vi "InitAll.vi"() -> (0 "error IO":errorcluster caption="error out")   [LabVIEW 2018]
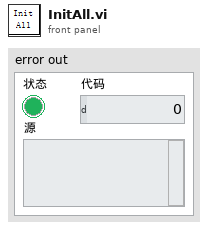
[diagram p1: front panel]
types:
  T1 = cluster{"Selected Index []":i32[], "Selected Items":string[]}
  T2 = enum16{"功率测量", "能量测量", "光谱测量", "时间波形", "偏振测量", "近远场"}
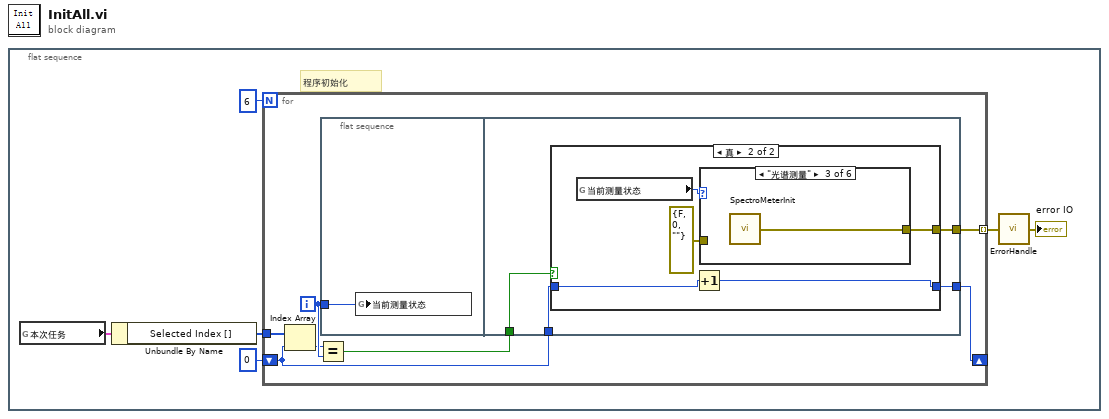
[diagram p0: block diagram]
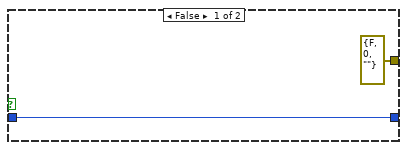
[diagram p2: hidden frame]
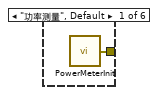
[diagram p3: hidden frame]
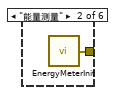
[diagram p4: hidden frame]
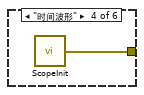
[diagram p5: hidden frame]
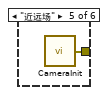
[diagram p6: hidden frame]
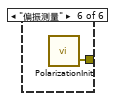
[diagram p7: hidden frame]
diagram:
  n1 = flat-sequence {
    frame #0 {
      # "程序初始化"
      n2 = global read "参数.vi" "本次任务"() -> (w2:T1)
      n3 = Unbundle By Name(w2) -> ("Selected Index []"=w1:i32[])
      n4 = for {
        N: 6 -> [_]
        tunnel: w1 -> [w13]
        shift-right: [w9] -> _
        shift-left: 0 -> [w7]
        tunnel: [w8] -> w4 mode=indexing
        i -> [w12]
        n5 = Index Array(array=w13, index=w7) -> (element=w10:i32)
        n6 = Equal?(x=w10, y=w12) -> (x = y?=w11:bool)
        n7 = flat-sequence {
          tunnel: w12 -> [w14]
          tunnel: w11 -> [w18]
          tunnel: w7 -> [w15]
          tunnel: [w17] -> w9
          tunnel: [w16] -> w8
          frame #0 {
            n8 = global write "参数.vi" "当前测量状态"(w14) -> ()
          }
          frame #1 {
            n9 = case shown="真" w18 {
              tunnel: w15 -> [w19 w21]
              tunnel: [w19 w25] -> w17
              tunnel: [errorcluster {"status"=FALSE, "code"=0, "source"=""} ("error out") w22] -> w16
              frame False {
              }
              frame True {
                n10 = global read "参数.vi" "当前测量状态"() -> (w24:T2)
                n11 = Increment(x=w21) -> (x+1=w25:i32)
                n12 = case shown="\"光谱测量\"" w24 {
                  tunnel: [w26 w27 w28 w29 w30 w31] -> w22
                  tunnel: errorcluster {"status"=FALSE, "code"=0, "source"=""} ("error out") -> [_ _ _ _ _ _]
                  frame "功率测量", Default {
                    n13 = call "PowerMeterInit.vi"() -> ("错误输出"=w26:errorcluster)  [unwired: 1 in]
                  }
                  frame "能量测量" {
                    n14 = call "EnergyMeterInit.vi"() -> ("错误输出"=w27:errorcluster)  [unwired: 1 in]
                  }
                  frame "光谱测量" {
                    n15 = call "SpectroMeterInit.vi"() -> ("error Out"=w28:errorcluster)  [unwired: 1 in]
                  }
                  frame "时间波形" {
                    n16 = call "ScopeInit.vi"() -> ("error out"=w29:errorcluster)  [unwired: 1 in]
                  }
                  frame "近远场" {
                    n17 = call "CameraInit.vi"() -> ("error out"=w30:errorcluster)  [unwired: 1 in]
                  }
                  frame "偏振测量" {
                    n18 = call "PolarizationInit.vi"() -> ("error IO 2"=w31:errorcluster)  [unwired: 3 in]
                  }
                }
              }
            }
          }
        }
      }
      n19 = call "ErrorHandle.vi"("Error"=w4) -> ("error IO"=→"error IO":errorcluster)
    }
  }
